vi "replaceComponent.vi"(0 "HGF_Composite":refnum<class "HGF_Composite.lvclass">, 1 "HGF_Component":refnum<class "HGF_Component.lvclass">, 2 "objectName":string, 3 "objectIndex":i32, 5 "error in (no error)":errorcluster) -> (14 "dup HGF_Composite":refnum<class "HGF_Composite.lvclass">, 19 "error out":errorcluster)   [LabVIEW 2014, in "HGF_BaseClasses.lvlib" / "HGF_Composite.lvclass"]
doc: "Replace a Component object within the Composite object.\n\nYou can specify either objectName or objectIndex.\nIf objectName is empty string the objectIndex will be used."
uses:
  HGF_Composite.lvclass
  HGF_Component/HGF_Component.lvclass
  HGF_Factory/HGF_Factory.lvclass
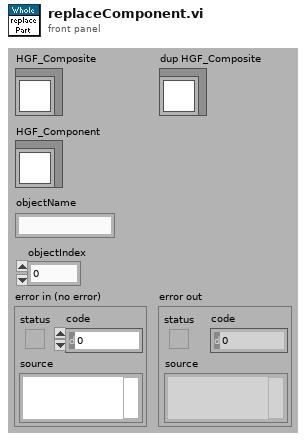
[diagram p1: front panel]
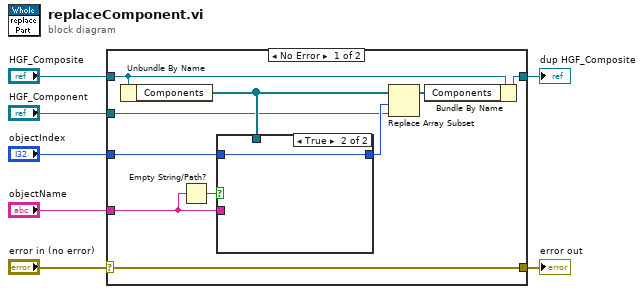
[diagram p0: block diagram]
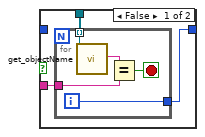
[diagram p2: hidden frame]
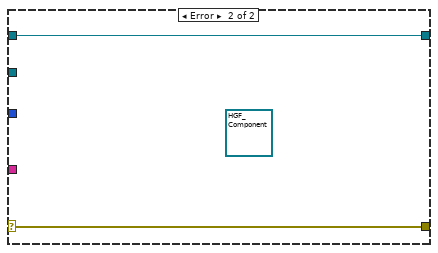
[diagram p3: hidden frame]
diagram:
  n1 = case shown="No Error" "error in (no error)" {
    selector: "error in (no error)" -> [w17 w28]
    tunnel: [w17 w28] -> w6
    tunnel: [w15 w27] -> w4
    tunnel: "HGF_Composite" -> [w16 w27]
    tunnel: "objectIndex" -> [w13 _]
    tunnel: "objectName" -> [w11 _]
    tunnel: "HGF_Component" -> [w8 _]
    frame No Error {
      n2 = Unbundle By Name(w16) -> ("Components"=w14:refnum<class "HGF_Component.lvclass">[])
      n3 = Empty String/Path?(string/path=w11) -> (empty?=w12:bool)
      n4 = case shown="True" w12 {
        tunnel: w14 -> [w20 _]
        tunnel: w11 -> [w19 _]
        tunnel: [w18 w26] -> w10
        tunnel: w13 -> [_ w26]
        frame False {
          n5 = for {
            tunnel: w20 -> [w25] mode=indexing
            tunnel: w19 -> [w22]
            tunnel: [w21] -> w18
            i -> [w21]
            stop <- w24 stop-if-true
            n6 = call "get_objectName.vi"("HGF_Factory"=w25) -> ("objectName"=w23:string)  [unwired: 1 in, 17 out]
            n7 = Equal?(x=w23, y=w22) -> (x = y?=w24:bool)
          }
        }
        frame True {
        }
      }
      n8 = Replace Array Subset(array=w14, new element=w8, index=w10) -> (w9:refnum<class "HGF_Component.lvclass">[])
      n9 = Bundle By Name(cluster=w16, "Components"=w9) -> (w15:refnum<class "HGF_Composite.lvclass">)
    }
    frame Error {
      (unwired) refnum<class "HGF_Component.lvclass"> refnum ("HGF_Component.lvclass")
    }
  }
  "error out" <- w6
  "dup HGF_Composite" <- w4
